vi "UI_Lubricate_Unit.vi"() -> ()   [LabVIEW 2014]
panel:
  out "DATA":T1
  in  "退出":bool
  # "试验单元监测参数"
  # "报警信息"
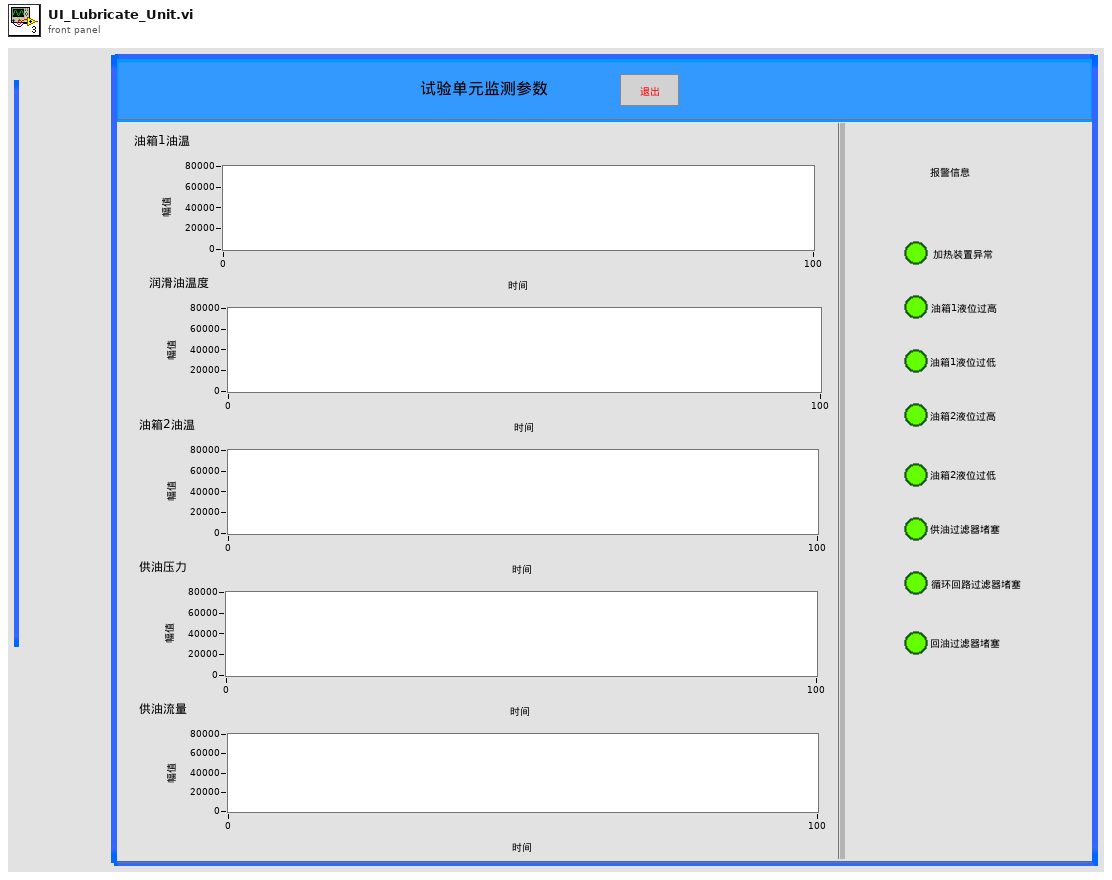
[diagram p1: front panel]
types:
  T1 = cluster{"油箱1油温 ":cluster{sgl, sgl, "油箱1油液温度":u16}, "润滑油温度":cluster{sgl, sgl, "润滑油温度":u16}, "油箱2油温":cluster{sgl, sgl, "油箱2油液温度":u16}, "径向液压缸加载压力 3":cluster{sgl, sgl, "试验轴承供油压力":u16}, "供油流量":cluster{sgl, sgl, "试验轴承供油流量":u16}, "报警信息":cluster{"试验轴承单元加热装置异常":bool, "试验轴承单元油箱1液位过高":bool, "试验轴承单元油箱1液位过低":bool, "试验轴承单元油箱2液位过高":bool, "试验轴承单元油箱2液位过低":bool, "试验轴承单元供油过滤器堵塞":bool, "试验轴承单元循环回路过滤器堵塞 2":bool, "试验轴承单元回油过滤器堵塞  ":bool}}
  T2 = cluster{"径向油缸加载压力":u16, "轴向油缸加载压力":u16, "油箱1油液温度":u16, "润滑油温度":u16, "油箱2油液温度":u16, "试验轴承供油压力":u16, "试验轴承供油流量":u16, "陪试轴承供油流量":u16, "陪试轴承供油压力":u16, "陪试轴承供油温度":u16, "液压子系统状态字":cluster{"加载单元":cluster{"供油过滤器堵塞报警":bool, "回油过滤器堵塞报警":bool, "液位过高报警":bool, "液位过低报警":bool}, "试验轴承单元":cluster{"加热装置异常报警":bool, "油箱1液位过高报警":bool, "油箱1液位过低报警":bool, "油箱2液位过高报警":bool, "油箱2液位过低报警":bool, "供油过滤器堵塞报警":bool, "循环回路过滤器堵塞报警":bool, "回油过滤器堵塞报警":bool}, "陪试轴承单元":cluster{"供油过滤器1堵塞报警":bool, "供油过滤器2堵塞报警":bool, "回油过滤器堵塞报警":bool, "油箱液位过高报警":bool, "油箱液位过低报警":bool}}}
  T3 = cluster{"加热装置异常报警":bool, "油箱1液位过高报警":bool, "油箱1液位过低报警":bool, "油箱2液位过高报警":bool, "油箱2液位过低报警":bool, "供油过滤器堵塞报警":bool, "循环回路过滤器堵塞报警":bool, "回油过滤器堵塞报警":bool}
  T4 = cluster{cluster{sgl, sgl, "油箱1油液温度":u16}, cluster{sgl, sgl, "润滑油温度":u16}, cluster{sgl, sgl, "油箱2油液温度":u16}, cluster{sgl, sgl, "试验轴承供油压力":u16}, cluster{sgl, sgl, "试验轴承供油流量":u16}, "试验轴承单元":cluster{"加热装置异常报警":bool, "油箱1液位过高报警":bool, "油箱1液位过低报警":bool, "油箱2液位过高报警":bool, "油箱2液位过低报警":bool, "供油过滤器堵塞报警":bool, "循环回路过滤器堵塞报警":bool, "回油过滤器堵塞报警":bool}}
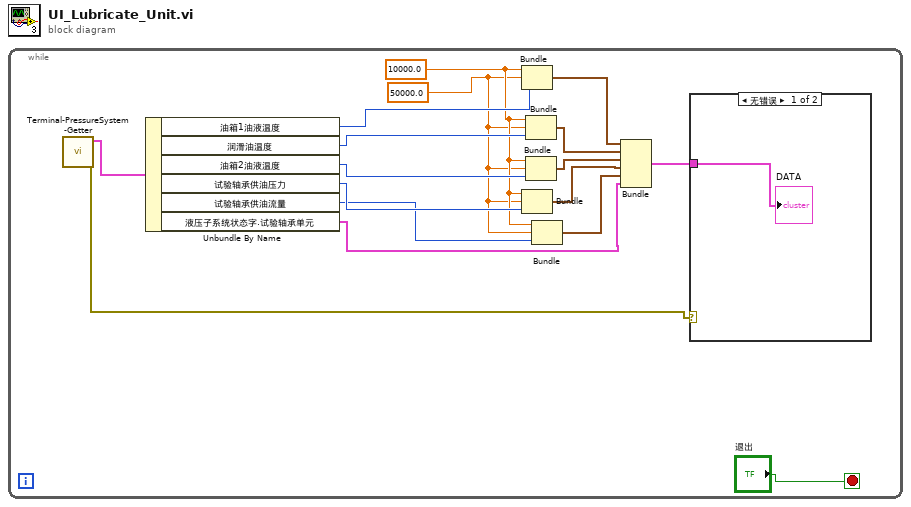
[diagram p0: block diagram]
diagram:
  n1 = while {
    stop <- "退出" stop-if-true
    w9 = sgl 50000.0
    w10 = sgl 10000.0
    n2 = call "Terminal-PressureSystem-Getter.vi"() -> ("error out"=w2:errorcluster, "设备信息"=w16:T2)  [unwired: 10 in]
    n3 = Unbundle By Name(w16) -> ("油箱1油液温度"=w15:u16, "润滑油温度"=w14:u16, "油箱2油液温度"=w13:u16, "试验轴承供油压力"=w12:u16, "试验轴承供油流量"=w11:u16, "液压子系统状态字.试验轴承单元"=w3:T3)
    n4 = Bundle(w10, w9, "油箱1油液温度"=w15) -> (w8:cluster{sgl, sgl, "油箱1油液温度":u16})  [unwired: 1 in]
    n5 = Bundle(w10, w9, "试验轴承供油压力"=w12) -> (w5:cluster{sgl, sgl, "试验轴承供油压力":u16})  [unwired: 1 in]
    n6 = Bundle(w10, w9, "润滑油温度"=w14) -> (w7:cluster{sgl, sgl, "润滑油温度":u16})  [unwired: 1 in]
    n7 = Bundle(w10, w9, "油箱2油液温度"=w13) -> (w6:cluster{sgl, sgl, "油箱2油液温度":u16})  [unwired: 1 in]
    n8 = Bundle(w10, w9, "试验轴承供油流量"=w11) -> (w4:cluster{sgl, sgl, "试验轴承供油流量":u16})  [unwired: 1 in]
    n9 = Bundle(w8, w7, w6, w5, w4, "试验轴承单元"=w3) -> (w1:T4)  [unwired: 1 in]
    n10 = case shown="无错误" w2 {
      tunnel: w1 -> [w18 _]
      frame No Error {
        "DATA" <- w18
      }
      frame Error {
      }
    }
  }
